vi "colorconv.vi"(8 "Color 3":bool[](array[boolean]), 9 "Color 2":bool[](array[boolean]), 11 "Color 1":bool[](array[boolean])) -> (0 "output waveform 3":digitalwaveform(waveform)={"t0"=timestamp(0 s since 1904-01-01), "dt"=1.0, "Y"={"transitions"=[], "data"=[]}}, 1 "output waveform 2":digitalwaveform(waveform)={"t0"=timestamp(0 s since 1904-01-01), "dt"=1.0, "Y"={"transitions"=[], "data"=[]}}, 3 "output waveform":digitalwaveform(waveform)={"t0"=timestamp(0 s since 1904-01-01), "dt"=1.0, "Y"={"transitions"=[], "data"=[]}})   [LabVIEW 2026]
uses:
  <vilib>/Waveform/DTblOps.llb/DTbl Boolean Array to Digital.vi
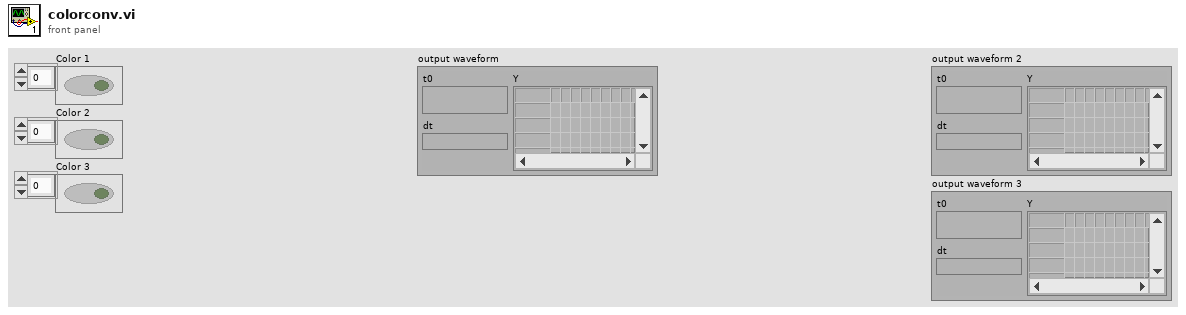
[diagram p1: front panel]
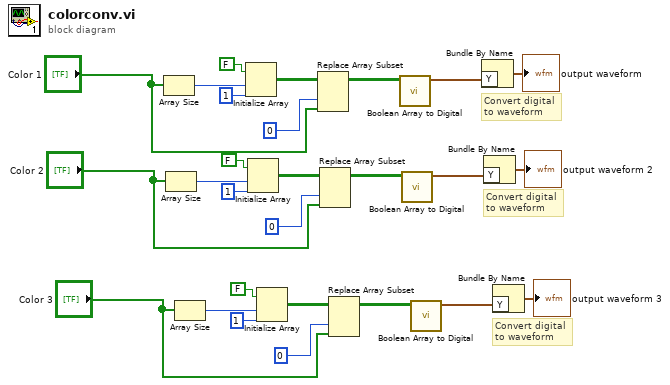
[diagram p0: block diagram]
diagram:
  # "Convert digital\nto waveform"
  # "Convert digital\nto waveform"
  # "Convert digital\nto waveform"
  n1 = Array Size(array="Color 1") -> (size(s)=w25:i32)
  n2 = Array Size(array="Color 2") -> (size(s)=w12:i32)
  n3 = Array Size(array="Color 3") -> (size(s)=w7:i32)
  n4 = Initialize Array(FALSE, w25, 1 ("dimension size")) -> (w24:bool[][])
  n5 = Initialize Array(FALSE, w12, 1 ("dimension size")) -> (w13:bool[][])
  n6 = Initialize Array(FALSE, w7, 1 ("dimension size")) -> (w6:bool[][])
  n7 = Replace Array Subset(array=w24, new element="Color 1", index (col)=0 ("index (row)")) -> (w27:bool[][])  [unwired: 1 in]
  n8 = Replace Array Subset(array=w13, new element="Color 2", index (col)=0 ("index (row)")) -> (w10:bool[][])  [unwired: 1 in]
  n9 = Replace Array Subset(array=w6, new element="Color 3", index (col)=0 ("index (row)")) -> (w9:bool[][])  [unwired: 1 in]
  n10 = call-poly <vilib>:"Boolean Array to Digital.vi"("boolean array"=w27) -> ("digital data"=w26:digitaldata)  [unwired: 3 in, 7 out]
  n11 = call-poly <vilib>:"Boolean Array to Digital.vi"("boolean array"=w10) -> ("digital data"=w11:digitaldata)  [unwired: 3 in, 7 out]
  n12 = call-poly <vilib>:"Boolean Array to Digital.vi"("boolean array"=w9) -> ("digital data"=w8:digitaldata)  [unwired: 3 in, 7 out]
  n13 = Bundle By Name("Y"=w26) -> (→"output waveform":digitalwaveform)  [unwired: 1 in]
  n14 = Bundle By Name("Y"=w11) -> (→"output waveform 2":digitalwaveform)  [unwired: 1 in]
  n15 = Bundle By Name("Y"=w8) -> (→"output waveform 3":digitalwaveform)  [unwired: 1 in]
